vi "Add Subfigure Letter.vi"(7 "Text":string="F", 8 "error in (no error)":errorcluster, 9 "Y Position":dbl, 10 "X Position":dbl, 11 "Plot ID in":T1 format="%x") -> (0 "error out":errorcluster, 3 "Plot ID Out":T1 format="%x")   [LabVIEW 2020]
uses:
  <vilib>/Heliosphere Research LLC/Advanced Plotting Toolkit/typedefs/PlotID.ctl
  <vilib>/Heliosphere Research LLC/Advanced Plotting Toolkit/api_annotations/TextProperties.ctl
  <vilib>/Heliosphere Research LLC/Advanced Plotting Toolkit/properties/Text.ctl
  <vilib>/Heliosphere Research LLC/Advanced Plotting Toolkit/typedefs/PlotColor.ctl
  <vilib>/Heliosphere Research LLC/Advanced Plotting Toolkit/properties/Text_FontSize.ctl
  <vilib>/Heliosphere Research LLC/Advanced Plotting Toolkit/properties/Text_FontStyle.ctl
  <vilib>/Heliosphere Research LLC/Advanced Plotting Toolkit/properties/Display.ctl
  <vilib>/Heliosphere Research LLC/Advanced Plotting Toolkit/Advanced Plotting Toolkit.lvlib
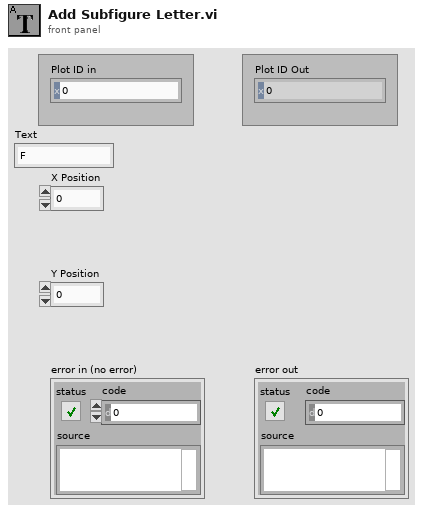
[diagram p1: front panel]
types:
  T1 = typedef "Advanced Plotting Toolkit.lvlib/PlotID.ctl" = i32
  T2 = typedef "Advanced Plotting Toolkit.lvlib/TextProperties.ctl" = cluster{"Text":T3, "Display":T7}
  T3 = typedef "Advanced Plotting Toolkit.lvlib/Text.ctl" = cluster{"Color":T4, "Background Color":T4, "Font Size (points)":T5, "Font Style":T6, "Rotation Angle":dbl}
  T4 = typedef "Advanced Plotting Toolkit.lvlib/PlotColor.ctl" = u32
  T5 = typedef "Advanced Plotting Toolkit.lvlib/Text_FontSize.ctl" = i32
  T6 = typedef "Advanced Plotting Toolkit.lvlib/Text_FontStyle.ctl" = enum16{"Automatic", "Normal", "Italic", "Bold"}
  T7 = typedef "Advanced Plotting Toolkit.lvlib/Display.ctl" = cluster{"Alpha":dbl, "Z Order":dbl}
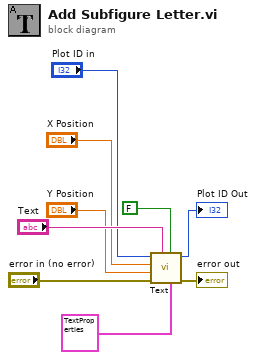
[diagram p0: block diagram]
diagram:
  n1 = call <vilib>:"Text.vi"("Properties"=T2 {"Text"={"Color"=0, "Background Color"=2147483647, "Font Size (points)"=-7, "Font Style"=enum."Bold", "Rotation Angle"=nan}, "Display"={"Alpha"=nan, "Z Order"=nan}}, "Relative Coordinates"=FALSE, "Text"="Text", "error in (no error)"="error in (no error)", "Y Position"="Y Position", "X Position"="X Position", "Plot ID"="Plot ID in") -> ("error out"=→"error out":errorcluster, "Plot ID Out"=→"Plot ID Out":T1)  [unwired: 3 in]
